vi "Query Voltage.vi"(8 "error in (no error)":errorcluster, 11 "VISA resource name":refnum<visa-resource-name>) -> (0 "error out":errorcluster, 1 "internal voltage (V)":sgl, 2 "main battery voltage (V)":sgl, 3 "VISA resource name out":refnum<visa-resource-name>, 4 "DSUB voltage (V)":sgl, 5 "Voltages":T1)   [LabVIEW 2012, in "Roboteq.lvlib"]
uses:
  Roboteq.lvlib
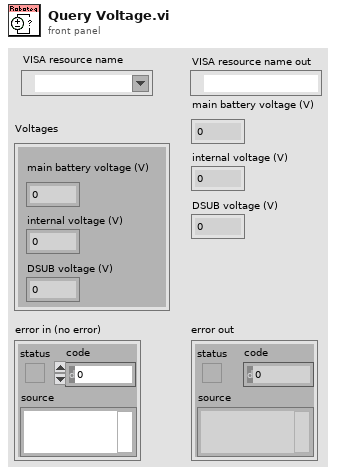
[diagram p1: front panel]
types:
  T1 = cluster{"main battery voltage (V)":sgl, "internal voltage (V)":sgl, "DSUB voltage (V)":sgl}
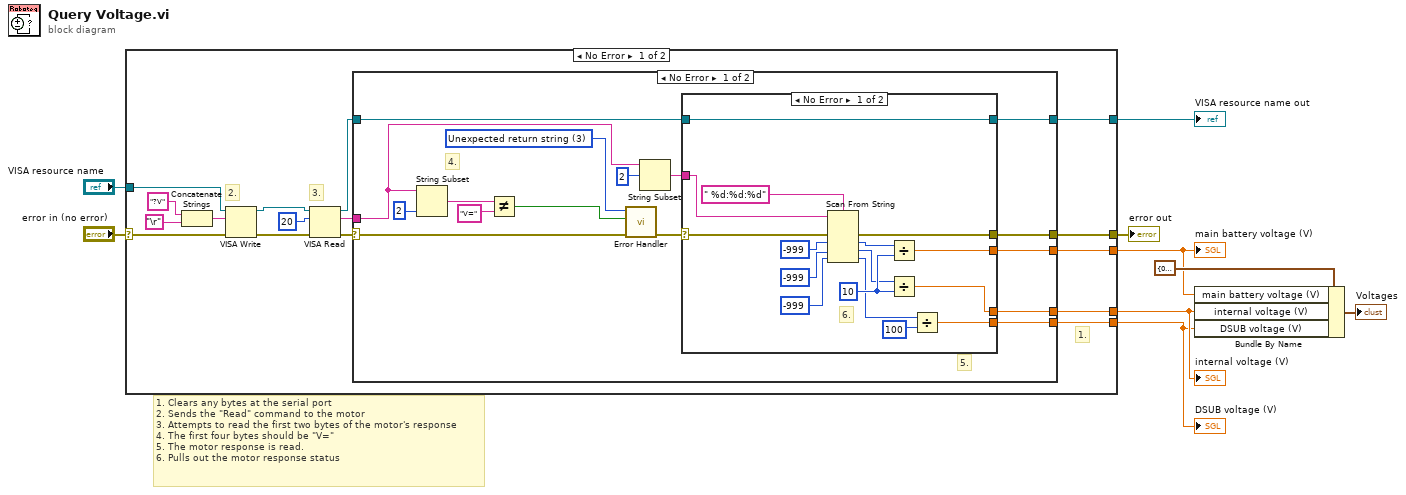
[diagram p0: block diagram]
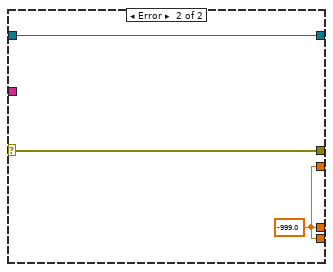
[diagram p2: hidden frame]
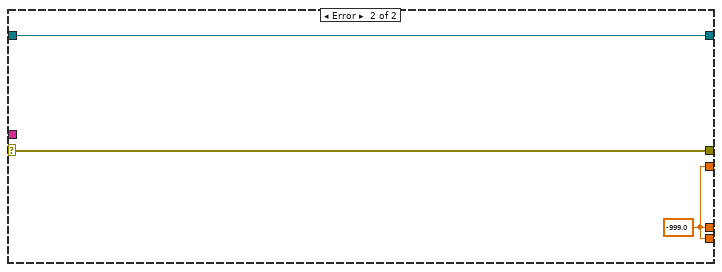
[diagram p3: hidden frame]
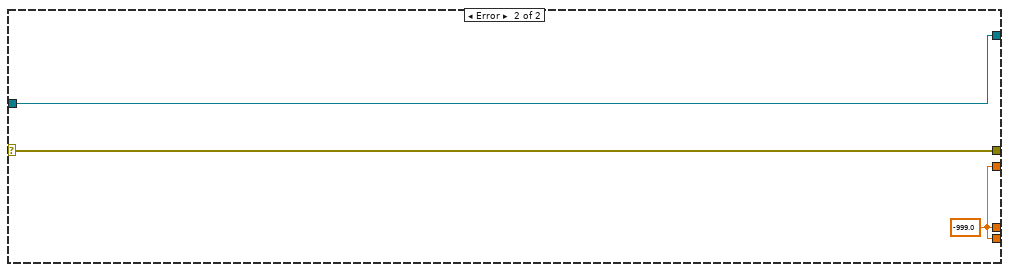
[diagram p4: hidden frame]
diagram:
  # "1. Clears any bytes at the serial port\n2. Sends the \"Read\" command to the motor\n3. Attempts to read the first two bytes of the motor's response\n4. The first four bytes should be \"V=\"\n5. The motor response is read.\n6. Pulls out the motor response status"
  n1 = case shown="No Error" "error in (no error)" {
    selector: "error in (no error)" -> [w10 w66]
    tunnel: [w13 w66] -> w8
    tunnel: [w15 w65] -> w2
    tunnel: [w14 w65] -> w1
    tunnel: [w16 w65] -> w3
    tunnel: "VISA resource name" -> [w11 w64]
    tunnel: [w12 w64] -> w6
    frame No Error {
      # "1."
      # "3."
      # "2."
      n2 = Concatenate Strings("?V" ("string"), "\r") -> (w24:string)
      n3 = VISA Write(VISA resource name=w11, write buffer=w24, error in (no error)=w10) -> (VISA resource name out=w21:refnum<visa-resource-name>, error out=w20:errorcluster)  [unwired: 1 out]
      n4 = VISA Read(VISA resource name=w21, byte count=u32 20, error in (no error)=w20) -> (VISA resource name out=w18:refnum<visa-resource-name>, read buffer=w17:string, error out=w19:errorcluster)  [unwired: 1 out]
      n5 = case shown="No Error" w19 {
        selector: w19 -> [w37 w63]
        tunnel: w17 -> [w28 _]
        tunnel: [w39 w63] -> w13
        tunnel: w18 -> [w41 w62]
        tunnel: [w40 w62] -> w12
        tunnel: [w33 w61] -> w16
        tunnel: [w32 w61] -> w15
        tunnel: [w31 w61] -> w14
        frame No Error {
          w34 = u16 3 items=["Scan timeout"=1, "Invalid motor checksum"=2, "Unexpected return string"=3, "Invalid address range"=4] ("Error type")
          # "5."
          # "4."
          n6 = String Subset(string=w28, length (rest)=2 ("length (rest)")) -> (substring=w29:string)  [unwired: 1 in]
          n7 = Not Equal?(x=w29, y="V=" ("string")) -> (x != y?=w36:bool)
          n8 = call "Error Handler.vi"("error in (no error)"=w37, "Error? (no error)"=w36, "Error type"=w34) -> ("error out"=w38:errorcluster)  [unwired: 8 in]
          n9 = String Subset(string=w28, offset (0)=2 ("length (rest)")) -> (substring=w26:string)  [unwired: 1 in]
          n10 = case shown="No Error" w38 {
            selector: w38 -> [w43 w60]
            tunnel: w26 -> [w44 _]
            tunnel: [w42 w60] -> w39
            tunnel: [w55 w59] -> w40
            tunnel: w41 -> [w55 w59]
            tunnel: [w54 w58] -> w33
            tunnel: [w53 w58] -> w32
            tunnel: [w52 w58] -> w31
            frame No Error {
              w57 = 10 ("y")
              # "6."
              n11 = Scan From String(format string=" %d:%d:%d", input string=w44, error in=w43, default 1=-999 ("default value 1"), default 2=-999 ("default value 1"), default 3=-999 ("default value 1")) -> (error out=w42:errorcluster, output 1=w48:i32, output 2=w47:i32, output 3=w46:i32)  [unwired: 1 in, 2 out]
              n12 = Divide(x=w48, y=w57) -> (x/y=w54:dbl)
              n13 = Divide(x=w47, y=w57) -> (x/y=w53:dbl)
              n14 = Divide(x=w46, y=100) -> (x/y=w52:dbl)
            }
            frame Error {
              w58 = sgl -999.0 ("main battery\nvoltage (V)")
            }
          }
        }
        frame Error {
          w61 = sgl -999.0 ("main battery\nvoltage (V)")
        }
      }
    }
    frame Error {
      w65 = sgl -999.0 ("main battery\nvoltage (V)")
    }
  }
  "VISA resource name out" <- w6
  "error out" <- w8
  "main battery voltage (V)" <- w3
  "internal voltage (V)" <- w2
  "DSUB voltage (V)" <- w1
  n15 = Bundle By Name(cluster=T1 {"main battery voltage (V)"=0.0, "internal voltage (V)"=0.0, "DSUB voltage (V)"=0.0} ("Voltages"), "main battery voltage (V)"=w3, "internal voltage (V)"=w2, "DSUB voltage (V)"=w1) -> (→"Voltages":T1)
